vi "setTimingProperties.vi"(8 "error in (no error)":errorcluster, 10 "Timing":T1, 11 "DigitalOutput.lvclass in":refnum<class "DigitalOutput.lvclass">) -> (0 "error out":errorcluster, 3 "DigitalOutput.lvclass out":refnum<class "DigitalOutput.lvclass">)   [LabVIEW 2009, in "Hardware.lvlib" / "Channels.lvlib" / "DigitalOutput.lvclass"]
uses:
  DigitalOutput.lvclass
  DigitalOutput.lvclass/DigitalOutput.ctl
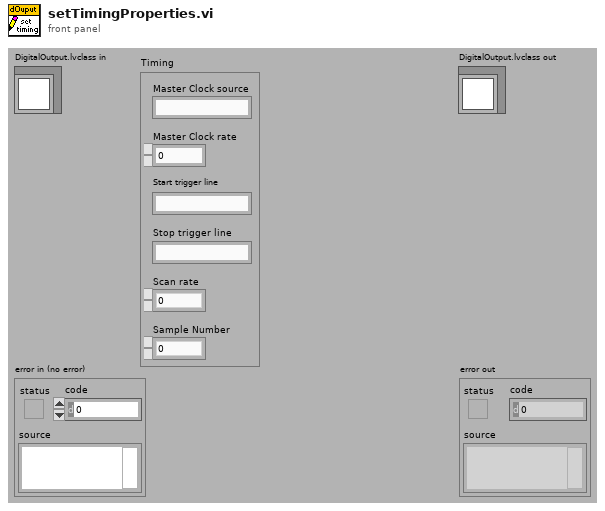
[diagram p1: front panel]
types:
  T1 = cluster{"Master Clock source":string, "Master Clock rate":dbl, "Start trigger line":string, "Scan rate":dbl, "Stop trigger line":string, "Sample Number":dbl}
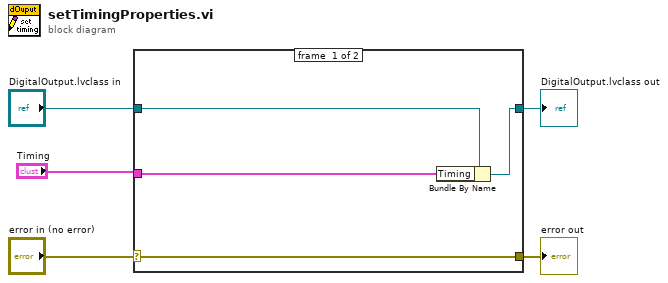
[diagram p0: block diagram]
diagram:
  n1 = case shown="No Error" "error in (no error)" {
    selector: "error in (no error)" -> [w9 w10]
    tunnel: [w9 w10] -> w4
    tunnel: [w7 w11] -> w2
    tunnel: "DigitalOutput.lvclass in" -> [w8 w11]
    tunnel: "Timing" -> [w6 _]
    frame #0 {
      n2 = Bundle By Name(cluster=w8, "Timing"=w6) -> (w7:refnum<class "DigitalOutput.lvclass">)
    }
    frame #1 {
    }
  }
  "error out" <- w4
  "DigitalOutput.lvclass out" <- w2
